vi "Build Send.vi"(8 "error in (no error)":errorcluster, 10 "Send VI":refnum<vi>, 11 "CS++Actor in":refnum<class "CS++Actor.lvclass">) -> (0 "error out":errorcluster, 3 "CS++Actor out":refnum<class "CS++Actor.lvclass">)   [LabVIEW 2014, in "CS++Actor.lvlib" / "CS++Actor.lvclass"]
doc: "Creates the send.vi of the new message."
uses:
  CS++Actor.lvclass
  CS++Actor.lvclass/CS++Actor.ctl
  <vilib>/Utility/traverseref.llb/TRef TravTarget.ctl
  <vilib>/Utility/traverseref.llb/VI Scripting - Traverse.lvlib
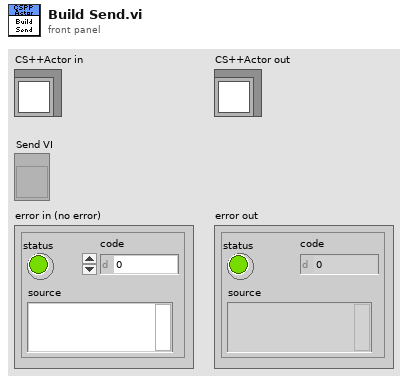
[diagram p1: front panel]
types:
  T1 = typedef "TRef TravTarget.ctl" = enum16{"FP", "BD", "Other"}
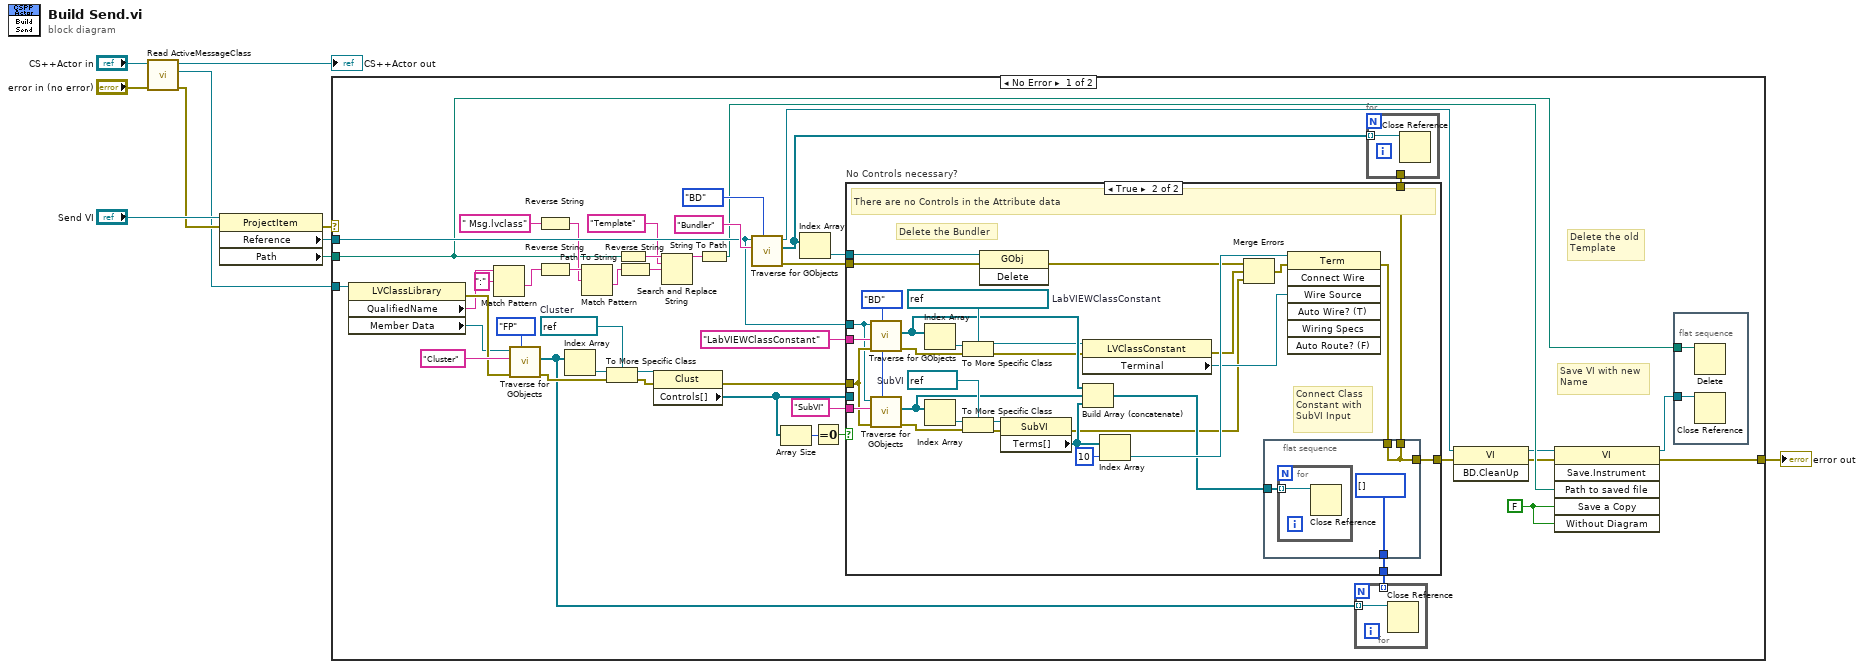
[diagram p0: block diagram]
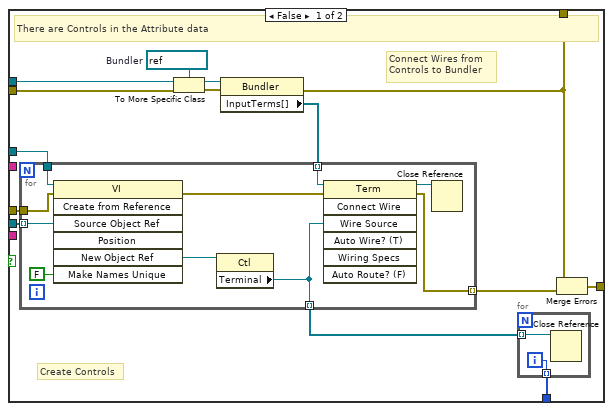
[diagram p2: hidden frame]
diagram:
  n1 = call "Read ActiveMessageClass.vi"("error in (no error)"="error in (no error)", "CS++Actor in"="CS++Actor in") -> ("error out"=w2:errorcluster, "ActiveMessageClass"=w1:refnum<vi>, "CS++Actor out"=→"CS++Actor out":refnum<class "CS++Actor.lvclass">)  [unwired: 7 in]
  n2 = property class="ProjectItem"(reference="Send VI", error in=w2) -> (error out=w9:errorcluster, "Reference"=w8:refnum<vi>, "Path"=w6:path)  [unwired: 1 out]
  n3 = case shown="No Error" w9 {
    selector: w9 -> [_ w122]
    tunnel: [w21 w122] -> w10
    tunnel: w1 -> [w55 _]
    tunnel: w8 -> [w38 _]
    tunnel: w6 -> [w23 _]
    frame No Error {
      w37 = FALSE ("Save a Copy")
      w51 = refnum<vi> refnum  # Cluster
      # "Delete the old\nTemplate"
      # "Save VI with new\nName"
      n4 = property class="LVClassLibrary"(reference=w55) -> (error out=w49:errorcluster, "QualifiedName"=w31:string, "Member Data"=w32:refnum<vi>)  [unwired: 1 in, 1 out]
      n5 = Match Pattern(string=w31, regular expression=":") -> (after substring=w24:string)  [unwired: 1 in, 3 out]
      n6 = call <vilib>:"Traverse for GObjects.vi"("Traverse Target"=TRef_TravTarget."FP", "error in (no error)"=w49, "Class Name"="Cluster" ("name/order"), "VI Refnum"=w32) -> ("error out"=w50:errorcluster, "References"=w41:refnum<vi>[])  [unwired: 4 in, 2 out]
      n7 = Reverse String(1:" Msg.lvclass" ("search string")) -> (0:w26:string)
      n8 = Reverse String(1:w24) -> (0:w28:string)
      n9 = Index Array(array=w41) -> (element=w52:refnum<vi>)  [unwired: 1 in]
      n10 = Match Pattern(string=w28, regular expression=w26) -> (after substring=w27:string)  [unwired: 1 in, 3 out]
      n11 = To More Specific Class(target class=w51, reference=w52, error in=w50) -> (specific class reference=w48:refnum<vi>, error out=w47:errorcluster)
      n12 = Path To String(path=w23) -> (string=w36:string)
      n13 = Reverse String(1:w27) -> (0:w29:string)
      n14 = property class="Clust"(reference=w48, error in=w47) -> (error out=w46:errorcluster, "Controls[]"=w16:refnum<vi>[])  [unwired: 1 out]
      n15 = Search and Replace String(input string=w36, search string="Template", replace string=w29) -> (result string=w34:string)  [unwired: 5 in, 3 out]
      n16 = String To Path(string=w34) -> (path=w33:path)
      n17 = call <vilib>:"Traverse for GObjects.vi"("Traverse Target"=TRef_TravTarget."BD", "Class Name"="Bundler", "VI Refnum"=w38) -> ("error out"=w43:errorcluster, "References"=w40:refnum<vi>[], "dup VI Refnum"=w20:refnum<vi>)  [unwired: 5 in, 1 out]
      n18 = Array Size(array=w16) -> (size(s)=w15:i32)
      n19 = Index Array(array=w40) -> (element=w14:refnum<vi>)  [unwired: 1 in]
      n20 = Equal To 0?(x=w15) -> (x = 0?=w13:bool)
      n21 = case "No Controls necessary?" shown="True" w13 {
        tunnel: w46 -> [w69 w102]
        tunnel: w43 -> [w68 w112]
        tunnel: [w61 w109] -> w42
        tunnel: [w60 w110] -> w39
        tunnel: w38 -> [w59 w101]
        tunnel: [w58 w111] -> w18
        tunnel: w16 -> [w57 _]
        tunnel: w14 -> [w56 w113]
        tunnel: "LabVIEWClassConstant" ("Class Name") -> [_ w108]
        tunnel: "SubVI" ("Class Name") -> [_ w103]
        frame False {
          w67 = refnum<vi> refnum  # Bundler
          # "Connect Wires from\nControls to Bundler"
          # "Create Controls"
          # "There are Controls in the Attribute data"
          n22 = To More Specific Class(target class=w67, reference=w56, error in=w68) -> (specific class reference=w66:refnum<vi>, error out=w65:errorcluster)
          n23 = property class="Bundler"(reference=w66, error in=w65) -> (error out=w60:errorcluster, "InputTerms[]"=w64:refnum<vi>[])  [unwired: 1 out]
          n24 = for {
            tunnel: w57 -> [w81] mode=indexing
            tunnel: w59 -> [w79]
            tunnel: w69 -> [w78]
            tunnel: w64 -> [w76] mode=indexing
            tunnel: [w75] -> w63 mode=indexing
            tunnel: [w73] -> w62 mode=indexing
            n25 = invoke class="VI" method="Create from Reference"(reference=w79, error in=w78, "Source Object Ref"=w81, "Make Names Unique"=FALSE ("Make Names Unique (F)")) -> (error out=w77:errorcluster, "New Object Ref"=w74:refnum<vi>)  [unwired: 3 in, 5 out]
            n26 = property class="Ctl"(reference=w74) -> ("Terminal"=w73:refnum<vi>)  [unwired: 1 in, 2 out]
            n27 = invoke class="Term" method="Connect Wire"(reference=w76, error in=w77, "Wire Source"=w73) -> (reference out=w72:refnum<vi>, error out=w75:errorcluster)  [unwired: 4 in, 5 out]
            n28 = Close Reference(reference=w72) -> ()  [unwired: 1 in, 1 out]
          }
          n29 = for {
            tunnel: w62 -> [w71] mode=indexing
            tunnel: [w70] -> w61 mode=indexing
            i -> [w70]
            n30 = Close Reference(reference=w71) -> ()  [unwired: 1 in, 1 out]
          }
          n31 = Merge Errors(w60, w63) -> (w58:errorcluster)
        }
        frame True {
          w98 = refnum<vi> refnum  # SubVI
          w106 = refnum<vi> refnum  # LabVIEWClassConstant
          w104 = TRef_TravTarget."BD" ("Traverse Target")
          # "Connect Class\nConstant with\nSubVI Input"
          # "Delete the Bundler"
          # "There are no Controls in the Attribute data"
          n32 = call <vilib>:"Traverse for GObjects.vi"("Traverse Target"=w104, "error in (no error)"=w102, "Class Name"=w108, "VI Refnum"=w101) -> ("error out"=w105:errorcluster, "References"=w90:refnum<vi>[])  [unwired: 4 in, 2 out]
          n33 = call <vilib>:"Traverse for GObjects.vi"("Traverse Target"=w104, "error in (no error)"=w102, "Class Name"=w103, "VI Refnum"=w101) -> ("error out"=w99:errorcluster, "References"=w89:refnum<vi>[])  [unwired: 4 in, 2 out]
          n34 = Index Array(array=w90) -> (element=w107:refnum<vi>)  [unwired: 1 in]
          n35 = Index Array(array=w89) -> (element=w100:refnum<vi>)  [unwired: 1 in]
          n36 = To More Specific Class(target class=w106, reference=w107, error in=w105) -> (specific class reference=w86:refnum<vi>, error out=w84:errorcluster)
          n37 = To More Specific Class(target class=w98, reference=w100, error in=w99) -> (specific class reference=w97:refnum<vi>, error out=w96:errorcluster)
          n38 = invoke class="GObj" method="Delete"(reference=w113, error in=w112) -> (error out=w93:errorcluster)  [unwired: 1 in, 2 out]
          n39 = property class="SubVI"(reference=w97, error in=w96) -> (error out=w82:errorcluster, "Terms[]"=w88:refnum<vi>[])  [unwired: 1 out]
          n40 = property class="LVClassConstant"(reference=w86, error in=w84) -> (error out=w83:errorcluster, "Terminal"=w85:refnum<vi>)  [unwired: 1 out]
          n41 = Build Array (concatenate)(w90, w89, w88) -> (w87:refnum<vi>[])
          n42 = Index Array(array=w88, index=10) -> (element=w94:refnum<vi>)
          n43 = Merge Errors(w93, w83, w82) -> (w92:errorcluster)
          n44 = flat-sequence {
            tunnel: [w114] -> w111
            tunnel: [w114] -> w110
            tunnel: [i32[] []] -> w109
            tunnel: w91 -> [w114]
            tunnel: w87 -> [w115]
            frame #0 {
              n45 = for {
                tunnel: w115 -> [w117] mode=indexing
                n46 = Close Reference(reference=w117) -> ()  [unwired: 1 in, 1 out]
              }
            }
          }
          n47 = invoke class="Term" method="Connect Wire"(reference=w94, error in=w92, "Wire Source"=w85) -> (error out=w91:errorcluster)  [unwired: 4 in, 6 out]
        }
      }
      n48 = for {
        tunnel: w41 -> [w121] mode=indexing
        tunnel: w42 -> [_] mode=indexing
        n49 = Close Reference(reference=w121) -> ()  [unwired: 1 in, 1 out]
      }
      n50 = for {
        tunnel: w40 -> [w120] mode=indexing
        tunnel: w39 -> [_]
        n51 = Close Reference(reference=w120) -> ()  [unwired: 1 in, 1 out]
      }
      n52 = invoke class="VI" method="BD.CleanUp"(reference=w20, error in=w18) -> (reference out=w19:refnum<vi>, error out=w17:errorcluster)  [unwired: 1 in, 1 out]
      n53 = invoke class="VI" method="Save.Instrument"(reference=w19, error in=w17, "Path to saved file"=w33, "Save a Copy"=w37, "Without Diagram"=w37) -> (reference out=w22:refnum<vi>, error out=w21:errorcluster)  [unwired: 1 in, 4 out]
      n54 = flat-sequence {
        tunnel: w22 -> [w119]
        tunnel: w23 -> [w118]
        frame #0 {
          n55 = Delete(path (use dialog)=w118) -> ()  [unwired: 4 in, 3 out]
          n56 = Close Reference(reference=w119) -> ()  [unwired: 1 in, 1 out]
        }
      }
    }
    frame Error {
    }
  }
  "error out" <- w10
